vi "TransformACoordinate.vi"(2 "Input":T2, 3 "C":T1, 4 "A":T1, 5 "B":T1) -> (0 "Result":T2, 1 "Ax + B":T1)   [LabVIEW 2011]
doc: "Performs the forward transformation of a point in the reference session to the current session coordinate system.\n\nReference point is passed to the routein in Input.[x2, y2, z2] \n\nInput.[x1,y1,z1] = A * (Input[x2,y2,z2] - C) + B\n\nThe output is the input vector and output vector in the pair of point structure. (i.e. the same point in two different coordinate systems).\n\nA is the rotation and scaling matrix, C is the offset vector to translate the reference point to a common point of rotation, B is the translation of the point to the current session coordinate system."
uses:
  Fiducial_pair.ctl
  <vilib>/Analysis/Matrix/Datatypes/RealMatrix.ctl
  <vilib>/Analysis/Matrix/Numeric/Conversions/Array To Matrix - RA.vi
  <vilib>/Analysis/Matrix/Numeric/Subtract/Subtract - RM,RM.vi
  <vilib>/Analysis/Matrix/Numeric/Multiply/Multiply - RM,RM.vi
  <vilib>/Analysis/Matrix/Numeric/Add/Add - RM,RM.vi
  <vilib>/Analysis/Matrix/NI_Matrix.lvlib
panel:
  # "A(x-c) = (y-b)"
  # "Fiducial Location Pair"
  # "Current Instrument Fiducial Location"
  # "Reference Instrument Fiducial Location"
  # "Fiducial Location Pair"
  # "Current Instrument Fiducial Location"
  # "Reference Instrument Fiducial Location"
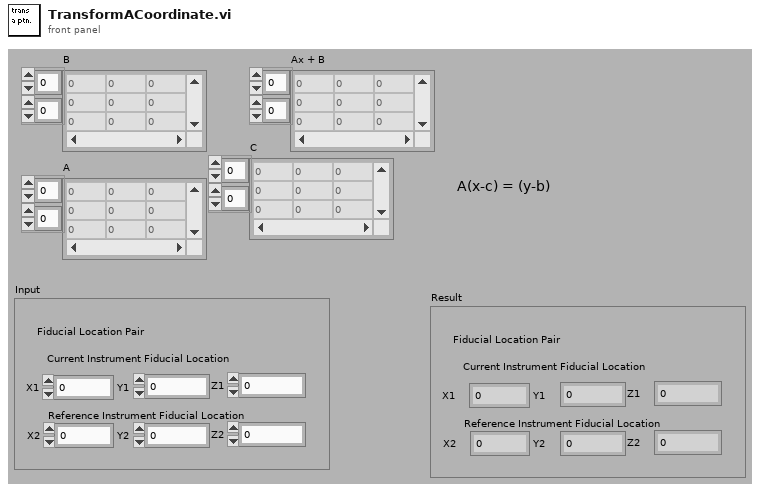
[diagram p1: front panel]
types:
  T1 = typedef "NI_Matrix.lvlib/RealMatrix.ctl" = dbl[][]
  T2 = typedef "Fiducial_pair.ctl" = cluster{"X1":dbl, "X2":dbl, "Y1":dbl, "Y2":dbl, "Z1":dbl, "Z2":dbl}
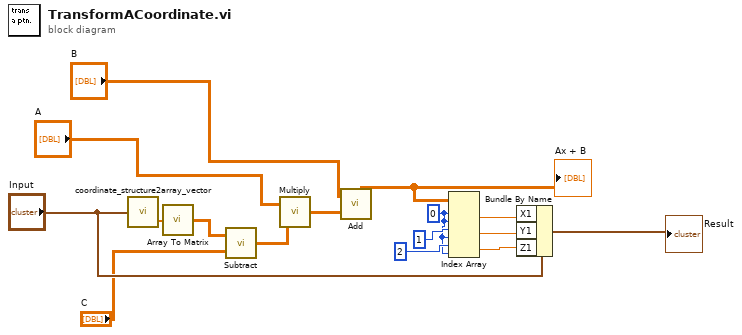
[diagram p0: block diagram]
diagram:
  w11 = 0 ("index (row)")
  n1 = call "coordinate_structure2array_vector.vi"("Fiducial_Pos_structure"="Input") -> ("Reference_Instrument_pos"=w7:dbl[])  [unwired: 1 out]
  n2 = call-poly <vilib>:"Array To Matrix.vi"("Real 1D Array"=w7) -> ("Real Matrix (Column Vector)"=w3:T1)
  n3 = call-poly <vilib>:"Subtract.vi"("Real Matrix B"="C", "Real Matrix A"=w3) -> ("A - B"=w1:T1)
  n4 = call-poly <vilib>:"Multiply.vi"("Real Matrix B"=w1, "Real Matrix A"="A") -> ("A * B"=w5:T1)
  n5 = call-poly <vilib>:"Add.vi"("Real Matrix B"=w5, "Real Matrix A"="B") -> ("A + B"=w9:T1)
  "Ax + B" <- w9
  n6 = Index Array(array=w9, index (row) #1=w11, index (col) #1=w11, index (row) #2=1 ("index (row)"), index (col) #2=w11, index (row) #3=2 ("index (row)"), index (col) #3=w11) -> (element #1=w10:dbl, element #2=w13:dbl, element #3=w15:dbl)
  n7 = Bundle By Name(cluster="Input", "X1"=w10, "Y1"=w13, "Z1"=w15) -> (→"Result":T2)
